vi "Read gRPC Configuration.vi"(8 "error in":errorcluster) -> (0 "error out":errorcluster, 1 "Manager Server Address":string, 2 "Plugin Server Address":string, 3 "Server Certificate File (.crt)":path, 4 "Local Manager Address":string, 5 "Server Key File (.key)":path)   [LabVIEW 2021, in "CIF Configuration File.lvlib"]
uses:
  CIF Configuration File.lvlib
  <vilib>/Utility/config.llb/Read Key (String).vi
  <vilib>/Utility/config.llb/Read Key (I32).vi
  <vilib>/Utility/config.llb/Read Key (Path).vi
  <vilib>/Utility/config.llb/NI_LVConfig.lvlib
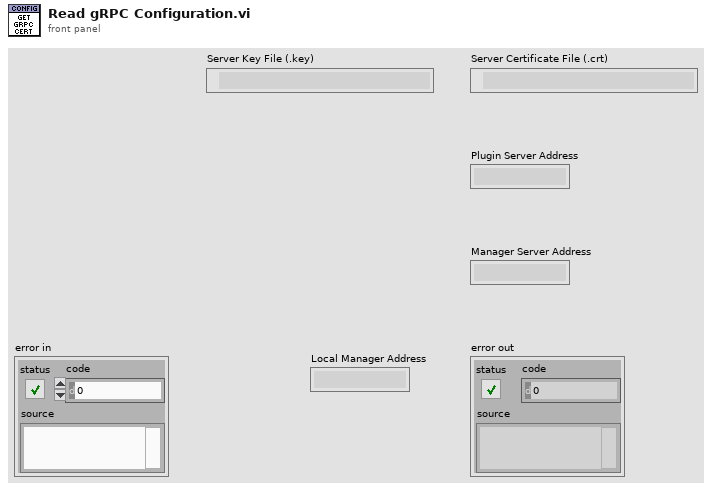
[diagram p1: front panel]
types:
  T1 = typedef "NI_LVConfig.lvlib/Config Data RefNum.ctl" = refnum<k1>
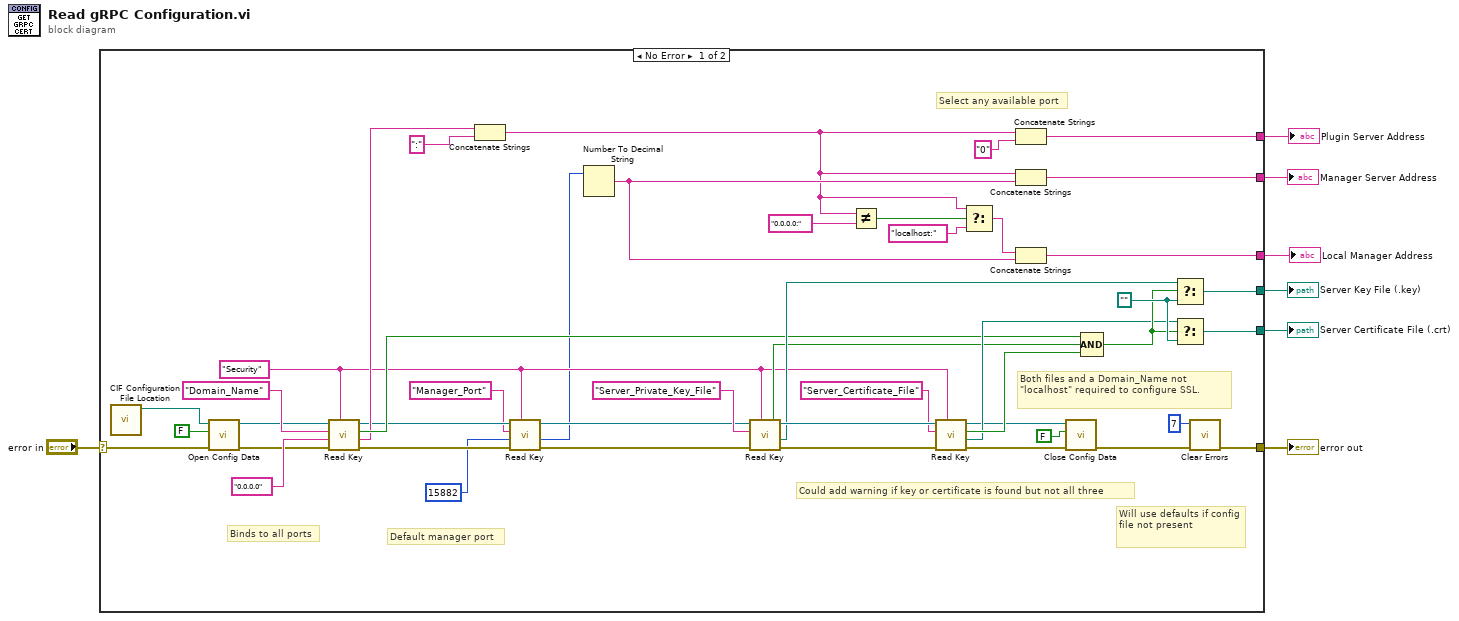
[diagram p0: block diagram]
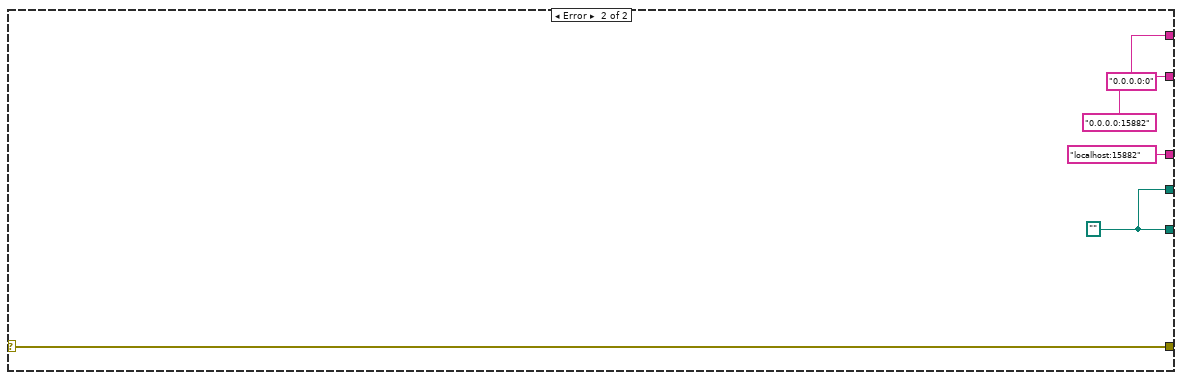
[diagram p2: hidden frame]
diagram:
  n1 = case shown="No Error" "error in" {
    selector: "error in" -> [w16 w58]
    tunnel: [w53 w57] -> w7
    tunnel: [w52 w57] -> w6
    tunnel: [w14 w58] -> w5
    tunnel: [w31 "0.0.0.0:15882"] -> w4
    tunnel: [w30 "0.0.0.0:0"] -> w3
    tunnel: [w17 "localhost:15882"] -> w2
    frame No Error {
      w47 = path ""
      w25 = "Security" ("Section")
      # "Will use defaults if config file not present"
      # "Could add warning if key or certificate is found but not all three"
      # "Select any available port"
      # "Default manager port"
      # "Binds to all ports"
      # "Both files and a Domain_Name not \"localhost\" required to configure SSL."
      n2 = call "CIF Configuration File Location.vi"() -> ("configuration file path"=w41:path)  [unwired: 11 in]
      n3 = call <vilib>:"Open Config Data.vi"("error in (no error)"=w16, "create file if necessary (T)"=FALSE, "configuration file path"=w41) -> ("error out"=w20:errorcluster, "refnum"=w19:T1)  [unwired: 6 in, 1 out]
      n4 = call-poly <vilib>:"Read Key.vi"("section"=w25, "error in (no error)"=w20, "default value"="0.0.0.0", "key"="Domain_Name", "refnum"=w19) -> ("error out"=w28:errorcluster, "value"=w33:string, "found?"=w34:bool, "refnum out"=w29:T1)  [unwired: 3 in]
      n5 = Concatenate Strings(w33, ":" ("string")) -> (w10:string)
      n6 = call-poly <vilib>:"Read Key.vi"("section"=w25, "error in (no error)"=w28, "default value"=15882, "key"="Manager_Port", "refnum"=w29) -> ("error out"=w26:errorcluster, "value"=w22:i32, "refnum out"=w27:T1)  [unwired: 3 in, 1 out]
      n7 = Number To Decimal String(number=w22) -> (decimal integer string=w18:string)  [unwired: 1 in]
      n8 = call-poly <vilib>:"Read Key.vi"("section"=w25, "error in (no error)"=w26, "key"="Server_Private_Key_File", "refnum"=w27) -> ("error out"=w50:errorcluster, "value"=w44:path, "found?"=w40:bool, "refnum out"=w48:T1)  [unwired: 4 in]
      n9 = Not Equal?(x=w10, y="0.0.0.0:") -> (x != y?=w11:bool)
      n10 = call-poly <vilib>:"Read Key.vi"("section"=w25, "error in (no error)"=w50, "key"="Server_Certificate_File", "refnum"=w48) -> ("error out"=w35:errorcluster, "value"=w43:path, "found?"=w46:bool, "refnum out"=w36:T1)  [unwired: 4 in]
      n11 = Select(t=w10, s=w11, f="localhost:" ("string")) -> (s? t:f=w8:string)
      n12 = Concatenate Strings(w10, "0" ("string")) -> (w30:string)
      n13 = Concatenate Strings(w10, w18) -> (w31:string)
      n14 = Concatenate Strings(w8, w18) -> (w17:string)
      n15 = call <vilib>:"Close Config Data.vi"("error in (no error)"=w35, "write file if changed (T)"=FALSE, "refnum"=w36) -> ("error out"=w15:errorcluster)  [unwired: 7 in, 1 out]
      n16 = Compound Arithmetic op=AND(w34, w40, w46) -> (w45:bool)
      n17 = Select(t=w44, s=w45, f=w47) -> (s? t:f=w52:path)
      n18 = Select(t=w43, s=w45, f=w47) -> (s? t:f=w53:path)
      n19 = call <vilib>:"Clear Errors.vi"("error in (no error)"=w15, "specific error code to clear (0: all)"=7) -> ("error out"=w14:errorcluster)  [unwired: 4 in, 1 out]
    }
    frame Error {
      w57 = path ""
    }
  }
  "error out" <- w5
  "Server Certificate File (.crt)" <- w7
  "Server Key File (.key)" <- w6
  "Manager Server Address" <- w4
  "Plugin Server Address" <- w3
  "Local Manager Address" <- w2
